vi "Add Square.vi"(8 "error in":errorcluster, 9 "Square":refnum<class "Square.lvclass">, 10 "Position":T1, 11 "Map in":refnum<class "Map.lvclass">) -> (0 "error out":errorcluster, 3 "Map out":refnum<class "Map.lvclass">)   [LabVIEW 2020, in "SquareBattle.lvlib" / "Map.lvclass"]
uses:
  Map.lvclass
  Position.ctl
  Square/Square.lvclass
  Map.lvclass/Map.ctl
  SquareBattle.lvlib
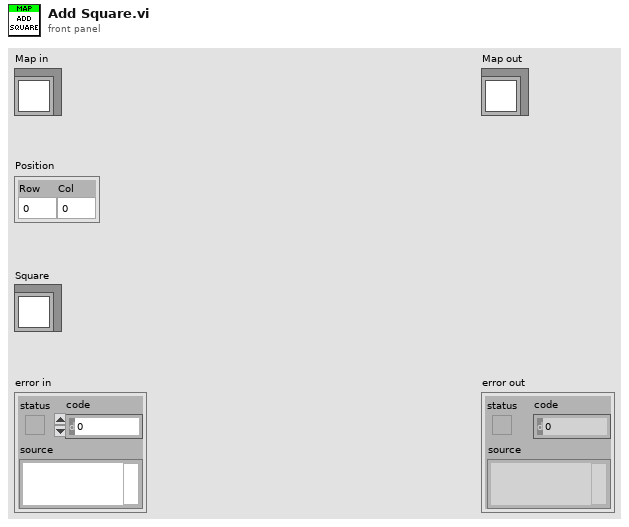
[diagram p1: front panel]
types:
  T1 = typedef "SquareBattle.lvlib/Position.ctl" = cluster{"Row":i32, "Col":i32}
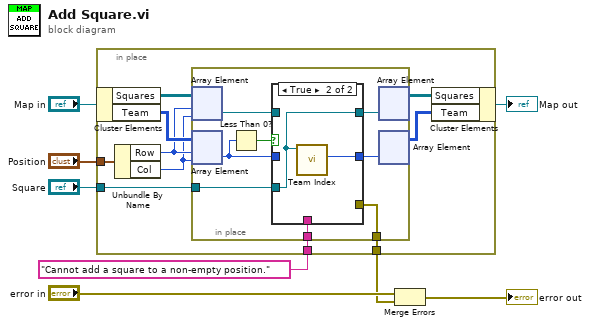
[diagram p0: block diagram]
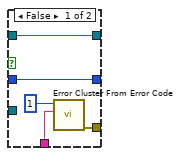
[diagram p2: hidden frame]
diagram:
  n1 = in-place {
    in-place-border: "Position" -> [w15]
    in-place-border: "Square" -> [w12]
    in-place-border: [w18] -> w6
    in-place-border: "Cannot add a square to a non-empty position." -> [w9]
    n2 = in-place-cluster #1("Map in") -> ("Squares"=w17:refnum<class "Square.lvclass">[][], "Team"=w16:i32[][])
    n3 = Unbundle By Name(w15) -> ("Row"=w14:i32, "Col"=w13:i32)
    n4 = in-place {
      in-place-border: w12 -> [w20]
      in-place-border: [w26] -> w18
      in-place-border: w9 -> [w19]
      n5 = in-place-array #2(w17, w14, w13) -> (w25:refnum<class "Square.lvclass">)
      n6 = in-place-array #3(w16, w14, w13) -> (w22:i32)
      n7 = Less Than 0?(x=w22) -> (x < 0?=w24:bool)
      n8 = case shown="True" w24 {
        tunnel: w25 -> [w30 _]
        tunnel: [w30 w32] -> w23
        tunnel: w22 -> [w29 _]
        tunnel: [w29 w33] -> w21
        tunnel: w20 -> [_ w32]
        tunnel: [w31 _] -> w26
        tunnel: w19 -> [w27 _]
        frame False {
          n9 = call <vilib>:"Error Cluster From Error Code.vi"("error message (\"\")"=w27, "error code (0)"=1) -> ("error out"=w31:errorcluster)  [unwired: 7 in]
        }
        frame True {
          n10 = call "Team Index.vi"("Square in"=w32) -> ("Team Index"=w33:i32)  [unwired: 10 in]
        }
      }
      n11 = in-place-array #2(w23) -> (w11:refnum<class "Square.lvclass">[][])  [unwired: 2 out]
      n12 = in-place-array #3(w21) -> (w10:i32[][])  [unwired: 2 out]
    }
    n13 = in-place-cluster #1("Squares"=w11, "Team"=w10) -> (→"Map out":refnum<class "Map.lvclass">)
  }
  n14 = Merge Errors("error in", w6) -> (→"error out":errorcluster)
